vi "Lockin.DAQ.getDAQState.vi"(8 "error in (no error)":errorcluster, 10 "state":T1=enum."created", 11 "Lockin.DAQ":refnum<class "Lockin.DAQ.lvclass">) -> (0 "error out":errorcluster, 3 "Lockin.DAQ":refnum<class "Lockin.DAQ.lvclass">)   [LabVIEW 2016, in "Lockin.DAQ.lvclass"]
doc: "---------------------------------------------------------------\nJKI State Machine Objects™\nhttp://jki.net/state-machine-objects/\nCopyright (C) 2005-2015, JKI <info@jki.net>\nALL RIGHTS RESERVEDJKI State Machine Objects (SMO) 1.0.0.4\nJKI - JKI\nCopyright (c) 2015, JKI"
uses:
  Lockin.DAQ.lvclass
  Typedefs/State-enum.ctl
  Lockin.DAQ.lvclass/Lockin.DAQ.ctl
panel:
  # "For instructions on how to use the JKI State Machine Objects, examples and video tutorials, visit:\nhttp://jki.net/state-machine-objects/\n\nJKI State Machine Objects™\nhttp://jki.net/state-machine-objects/\nCopyright (C) 2005-2015, JKI <info@jki.net>\nALL RIGHTS RESERVED"
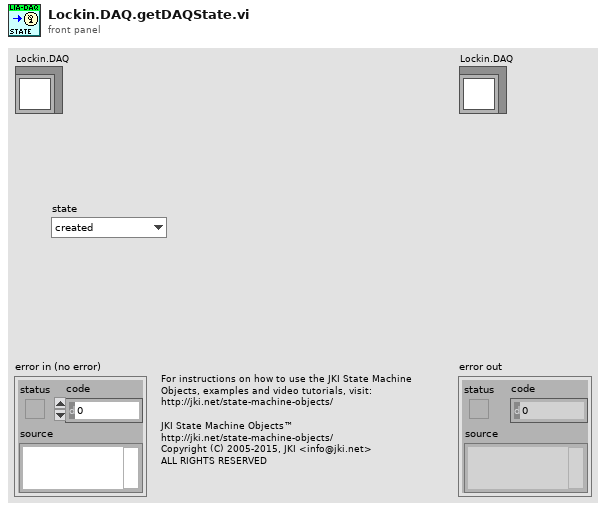
[diagram p1: front panel]
types:
  T1 = typedef "Lockin.DAQ.lvclass/State-enum.ctl" = enum16{"idle", "created", "started", "stopped", "sweeping"}
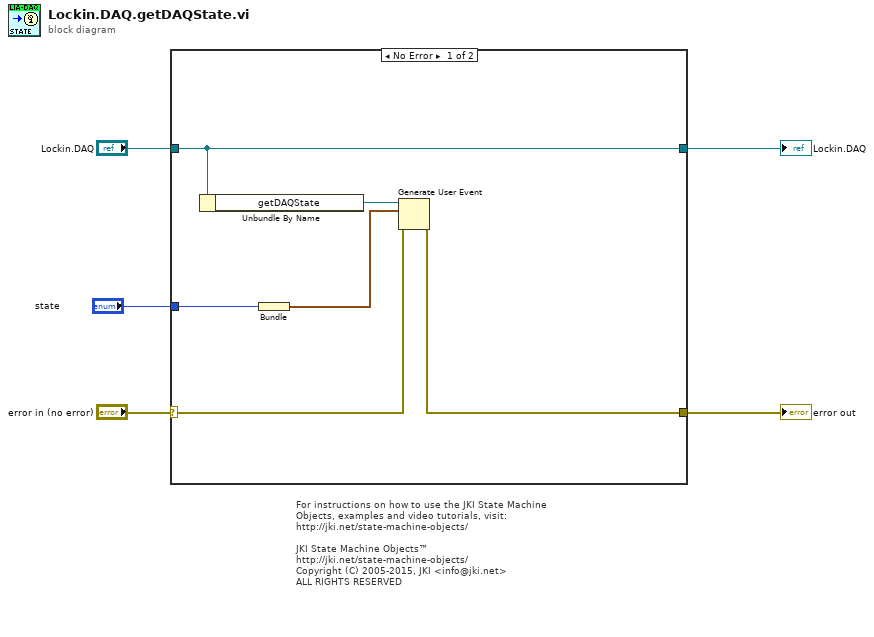
[diagram p0: block diagram]
diagram:
  # "For instructions on how to use the JKI State Machine Objects, examples and video tutorials, visit:\nhttp://jki.net/state-machine-objects/\n\nJKI State Machine Objects™\nhttp://jki.net/state-machine-objects/\nCopyright (C) 2005-2015, JKI <info@jki.net>\nALL RIGHTS RESERVED"
  n1 = case shown="No Error" "error in (no error)" {
    selector: "error in (no error)" -> [w11 w13]
    tunnel: [w8 w13] -> w4
    tunnel: [w7 w12] -> w5
    tunnel: "Lockin.DAQ" -> [w7 w12]
    tunnel: "state" -> [w10 _]
    frame No Error {
      n2 = Unbundle By Name(w7) -> ("getDAQState"=w9:refnum<user-event>)
      n3 = Bundle("state"=w10) -> (w6:cluster{"state":T1})  [unwired: 1 in]
      n4 = Generate User Event(user event=w9, event data cluster=w6, error in=w11) -> (error out=w8:errorcluster)  [unwired: 1 in, 1 out]
    }
    frame Error {
    }
  }
  "error out" <- w4
  "Lockin.DAQ" <- w5
